vi "Data Listener Repository.vi"(0 "Connection ID":u64, 1 "Action(ReadRepository)":T1(ring), 5 "error in (no error)":errorcluster) -> (9 "ProcessViRef":refnum<vi>, 11 "ProcessSyncQueue":refnum<queue>, 13 "FromProcessQueue":refnum<queue>, 15 "ToProcessQueue":refnum<queue>, 17 "ProcessAlreadyStarted":bool, 19 "error out":errorcluster)   [LabVIEW 2017, in "Front Panel Publisher.lvlib" / "Websocket.lvclass"]
uses:
  Websocket.lvclass
  Data Listener.ctl
panel:
  # "Use this indicator for sending messages to the Process VI"
  # "These indicators are used by the process VIs"
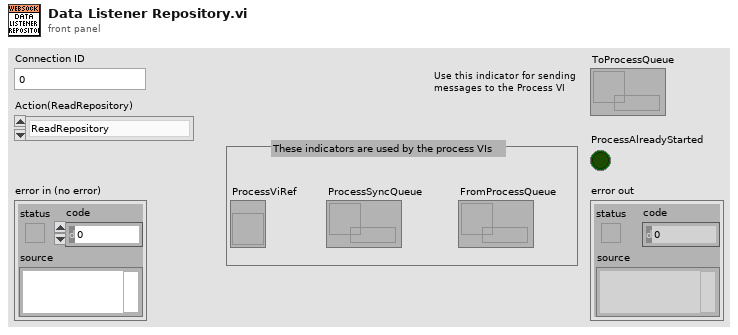
[diagram p1: front panel]
types:
  T1 = enum16{"ReadRepository", "CreateNew", "CreateOrLookUpExisting", "ReadRepositoryAndDestroy"}
  T2 = typedef "Front Panel Publisher.lvlib/Websocket.lvclass/Data Listener.ctl" = cluster{"ToProcessQueue":refnum<queue>, "FromProcessQueue":refnum<queue>, "ProcessSyncQueue":refnum<queue>, "ProcessViRef":refnum<vi>}
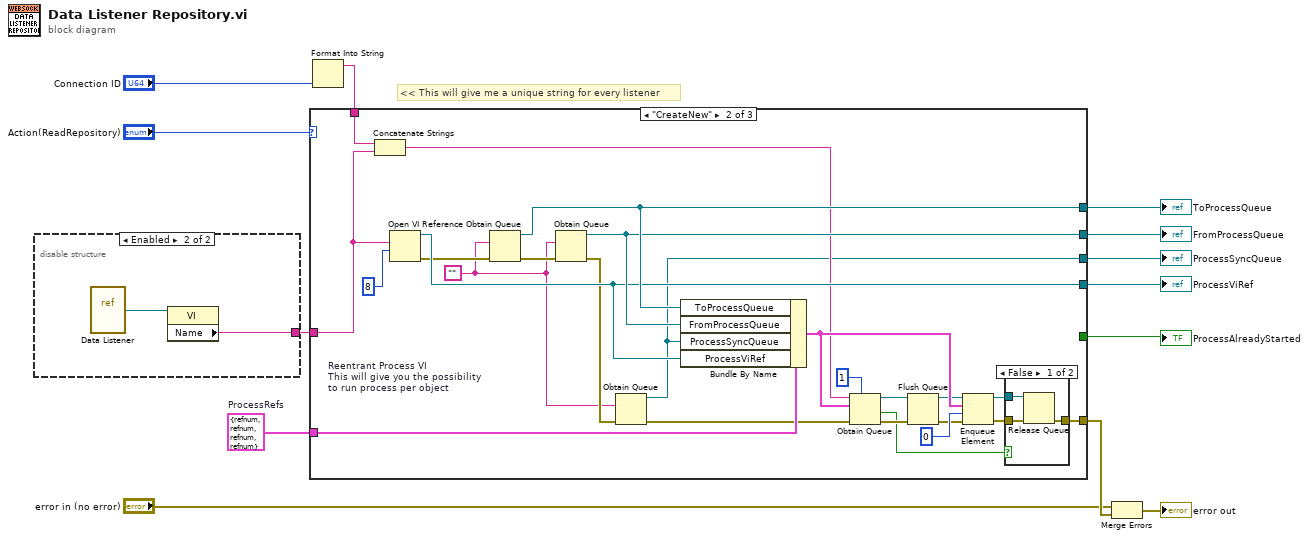
[diagram p0: block diagram]
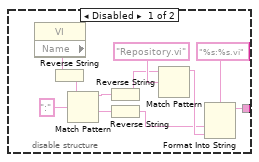
[diagram p2: hidden frame]
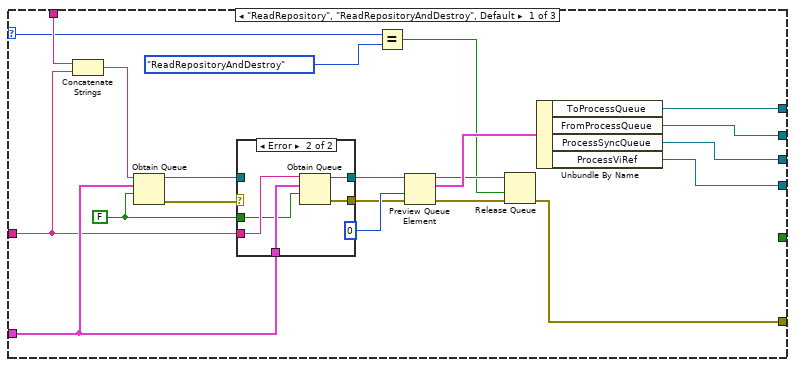
[diagram p3: hidden frame]
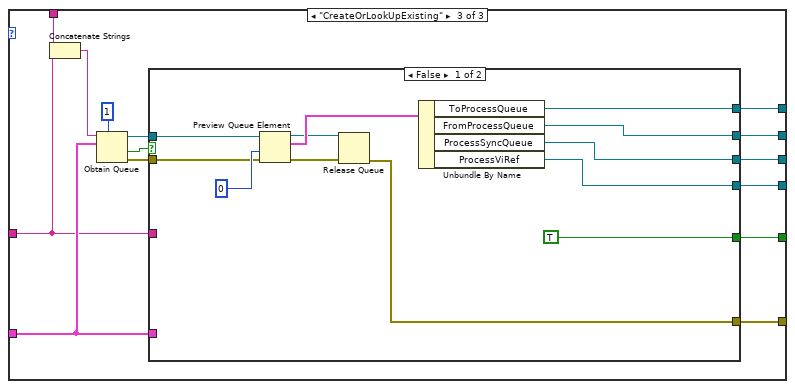
[diagram p6: hidden frame]
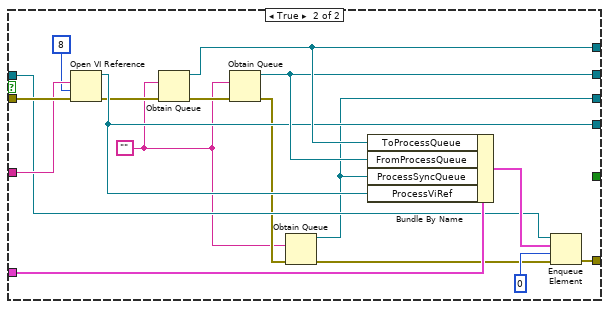
[diagram p7: hidden frame]
diagram:
  w8 = T2 {"ToProcessQueue"=refnum, "FromProcessQueue"=refnum, "ProcessSyncQueue"=refnum, "ProcessViRef"=refnum}  # ProcessRefs
  # "<< This will give me a unique string for every listener"
  n1 = disable-structure shown="Enabled" {
    disable-tunnel: [w14 w25] -> w5
    frame Disabled {
      n2 = property class="VI"() -> ("Name"=w16:string)  [unwired: 2 in, 2 out]
      n3 = Reverse String(1:w16) -> (0:w17:string)
      n4 = Match Pattern(string=w17, regular expression=":") -> (before substring=w21:string, after substring=w18:string)  [unwired: 1 in, 2 out]
      n5 = Reverse String(1:w21) -> (0:w22:string)
      n6 = Reverse String(1:w18) -> (0:w20:string)
      n7 = Match Pattern(string=w22, regular expression="Repository.vi") -> (before substring=w24:string)  [unwired: 1 in, 3 out]
      n8 = Format Into String(format string="%s:%s.vi", w20, w24) -> (resulting string=w14:string)  [unwired: 2 in, 1 out]
    }
    frame Enabled {
      n9 = vi-ref "Data Listener.vi"() -> (w26:refnum<vi>)
      n10 = property class="VI"(reference=w26) -> ("Name"=w25:string)  [unwired: 1 in, 2 out]
    }
  }
  n11 = Format Into String("Connection ID") -> (resulting string=w2:string)  [unwired: 3 in, 1 out]
  n12 = case shown="\"CreateNew\"" "Action(ReadRepository)" {
    selector: "Action(ReadRepository)" -> [w28 _ _]
    tunnel: [w42 w63 w95] -> w12
    tunnel: [w44 w79 w97] -> w10
    tunnel: [w43 w78 w96] -> w11
    tunnel: [w45 w77 w94] -> w9
    tunnel: w8 -> [w37 w69 w90]
    tunnel: w2 -> [w35 w68 w86]
    tunnel: [w30 w57 w93] -> w6
    tunnel: w5 -> [w34 w66 w85]
    tunnel: [_ _ w88] -> w4
    frame "ReadRepository", "ReadRepositoryAndDestroy", Default {
      w36 = FALSE ("create if not found? (T)")
      n13 = Concatenate Strings(w35, w34) -> (w33:string)
      n14 = Obtain Queue(name (unnamed)=w33, element data type=w37, create if not found? (T)=w36) -> (queue out=w39:refnum<queue>, error out=w41:errorcluster)  [unwired: 2 in, 1 out]
      n15 = case shown="Error" w41 {
        selector: w41 -> [w49 _]
        tunnel: [w49 w51] -> w40
        tunnel: w39 -> [w48 _]
        tunnel: [w48 w52] -> w38
        tunnel: w37 -> [_ w54]
        tunnel: w34 -> [_ w53]
        tunnel: w36 -> [_ w50]
        frame No Error {
        }
        frame Error {
          n16 = Obtain Queue(name (unnamed)=w53, element data type=w54, create if not found? (T)=w50) -> (queue out=w52:refnum<queue>, error out=w51:errorcluster)  [unwired: 2 in, 1 out]
        }
      }
      n17 = Equal?(x=w28, y=T1."ReadRepositoryAndDestroy") -> (x = y?=w27:bool)
      n18 = Preview Queue Element(queue=w38, timeout in ms (-1)=0, error in (no error)=w40) -> (queue out=w32:refnum<queue>, element=w46:T2, error out=w31:errorcluster)  [unwired: 1 out]
      n19 = Release Queue(queue=w32, force destroy? (F)=w27, error in (no error)=w31) -> (error out=w30:errorcluster)  [unwired: 2 out]
      n20 = Unbundle By Name(w46) -> ("ToProcessQueue"=w44:refnum<queue>, "FromProcessQueue"=w43:refnum<queue>, "ProcessSyncQueue"=w42:refnum<queue>, "ProcessViRef"=w45:refnum<vi>)
    }
    frame "CreateNew" {
      w74 = 8  # Reentrant Process VI This will give you the possibility to run process per object
      w55 = ""
      n21 = Concatenate Strings(w68, w66) -> (w67:string)
      n22 = Open VI Reference(vi path=w66, options=w74) -> (vi reference=w77:refnum<vi>, error out=w75:errorcluster)  [unwired: 4 in]
      n23 = Obtain Queue(element data type=w55, error in (no error)=w75) -> (queue out=w79:refnum<queue>, error out=w76:errorcluster)  [unwired: 3 in, 1 out]
      n24 = Obtain Queue(element data type=w55, error in (no error)=w76) -> (queue out=w78:refnum<queue>, error out=w65:errorcluster)  [unwired: 3 in, 1 out]
      n25 = Obtain Queue(element data type=w55, error in (no error)=w65) -> (queue out=w63:refnum<queue>, error out=w64:errorcluster)  [unwired: 3 in, 1 out]
      n26 = Bundle By Name(cluster=w69, "ToProcessQueue"=w79, "FromProcessQueue"=w78, "ProcessSyncQueue"=w63, "ProcessViRef"=w77) -> (w72:T2)
      n27 = Obtain Queue(max queue size (-1, unlimited)=1, name (unnamed)=w67, element data type=w72, error in (no error)=w64) -> (queue out=w73:refnum<queue>, created new?=w56:bool, error out=w61:errorcluster)  [unwired: 1 in]
      n28 = Flush Queue(queue=w73, error in (no error)=w61) -> (queue out=w62:refnum<queue>, error out=w60:errorcluster)  [unwired: 1 out]
      n29 = Enqueue Element(queue=w62, element=w72, timeout in ms (-1)=0, error in (no error)=w60) -> (queue out=w59:refnum<queue>, error out=w58:errorcluster)  [unwired: 1 out]
      n30 = case shown="False" w56 {
        tunnel: w58 -> [w82 w83]
        tunnel: w59 -> [w81 _]
        tunnel: [w80 w83] -> w57
        frame False {
          n31 = Release Queue(queue=w81, error in (no error)=w82) -> (error out=w80:errorcluster)  [unwired: 1 in, 2 out]
        }
        frame True {
        }
      }
    }
    frame "CreateOrLookUpExisting" {
      n32 = Concatenate Strings(w86, w85) -> (w84:string)
      n33 = Obtain Queue(max queue size (-1, unlimited)=1, name (unnamed)=w84, element data type=w90) -> (queue out=w91:refnum<queue>, created new?=w92:bool, error out=w89:errorcluster)  [unwired: 2 in]
      n34 = case shown="False" w92 {
        tunnel: [w109 w126] -> w97
        tunnel: [w108 w125] -> w96
        tunnel: [w107 w112] -> w95
        tunnel: [w106 w124] -> w94
        tunnel: [w98 w123] -> w93
        tunnel: w90 -> [_ w122]
        tunnel: w89 -> [w103 w117]
        tunnel: w85 -> [_ w116]
        tunnel: w91 -> [w104 w115]
        tunnel: [TRUE _] -> w88
        frame False {
          n35 = Preview Queue Element(queue=w104, timeout in ms (-1)=0, error in (no error)=w103) -> (queue out=w100:refnum<queue>, element=w102:T2, error out=w99:errorcluster)  [unwired: 1 out]
          n36 = Release Queue(queue=w100, error in (no error)=w99) -> (error out=w98:errorcluster)  [unwired: 1 in, 2 out]
          n37 = Unbundle By Name(w102) -> ("ToProcessQueue"=w109:refnum<queue>, "FromProcessQueue"=w108:refnum<queue>, "ProcessSyncQueue"=w107:refnum<queue>, "ProcessViRef"=w106:refnum<vi>)
        }
        frame True {
          w111 = ""
          n38 = Open VI Reference(vi path=w116, options=8, error in (no error)=w117) -> (vi reference=w124:refnum<vi>, error out=w120:errorcluster)  [unwired: 3 in]
          n39 = Obtain Queue(element data type=w111, error in (no error)=w120) -> (queue out=w126:refnum<queue>, error out=w121:errorcluster)  [unwired: 3 in, 1 out]
          n40 = Obtain Queue(element data type=w111, error in (no error)=w121) -> (queue out=w125:refnum<queue>, error out=w114:errorcluster)  [unwired: 3 in, 1 out]
          n41 = Obtain Queue(element data type=w111, error in (no error)=w114) -> (queue out=w112:refnum<queue>, error out=w113:errorcluster)  [unwired: 3 in, 1 out]
          n42 = Bundle By Name(cluster=w122, "ToProcessQueue"=w126, "FromProcessQueue"=w125, "ProcessSyncQueue"=w112, "ProcessViRef"=w124) -> (w119:T2)
          n43 = Enqueue Element(queue=w115, element=w119, timeout in ms (-1)=0, error in (no error)=w113) -> (error out=w123:errorcluster)  [unwired: 2 out]
        }
      }
    }
  }
  "ProcessSyncQueue" <- w12
  "ToProcessQueue" <- w10
  "FromProcessQueue" <- w11
  "ProcessViRef" <- w9
  "ProcessAlreadyStarted" <- w4
  n44 = Merge Errors("error in (no error)", w6) -> (→"error out":errorcluster)
